vi "crd_processWaveform.vi"(10 "No Avg.":i32, 11 "Queue in":refnum<queue>) -> (0 "error out":errorcluster, 1 "tau (us)":dbl, 2 "Decay":cluster{sgl[], "Best Exponential Fit":dbl[]}[](graph), 3 "Queue out":refnum<queue>)   [LabVIEW 2011]
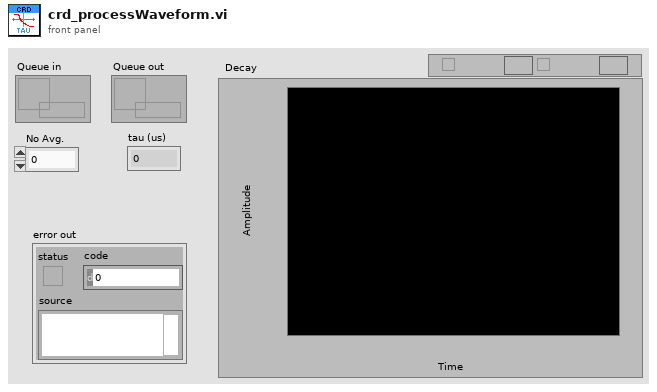
[diagram p1: front panel]
types:
  T1 = cluster{i32, "Sample Internal":sgl, "Data (Volts)":dbl[]}
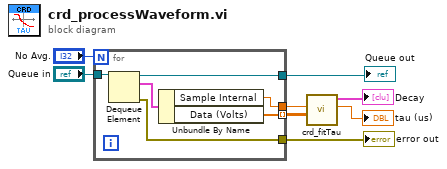
[diagram p0: block diagram]
diagram:
  n1 = for {
    N: "No Avg." -> [_]
    tunnel: [w14] -> w3
    tunnel: [w13] -> w4 mode=indexing
    tunnel: "Queue in" -> [w12]
    tunnel: [w11] -> w7
    tunnel: [w9] -> w8
    n2 = Dequeue Element(queue=w12) -> (queue out=w11:refnum<queue>, element=w10:T1, error out=w9:errorcluster)  [unwired: 2 in, 1 out]
    n3 = Unbundle By Name(w10) -> ("Sample Internal"=w14:sgl, "Data (Volts)"=w13:dbl[])
  }
  "error out" <- w8
  "Queue out" <- w7
  n4 = call "crd_fitTau.vi"("y Data (volts)"=w4, "Sample Internal"=w3) -> ("tau (us)"=→"tau (us)":dbl, "Decay"=→"Decay":cluster{sgl[], "Best Exponential Fit":dbl[]}[])  [unwired: 8 in]
